vi "SortGraphIndex.vi"(4 "Error In":errorcluster, 7 "ConfigurationTotale":T2) -> (0 "Error Out":errorcluster, 3 "GraphIndex":T1)   [LabVIEW 2017]
uses:
  DefDeType/ConfigTotale.ctl
  DefDeType/VoltageChannels.ctl
  DefDeType/WBridgeChannels.ctl
  DefDeType/Configuration.ctl
panel:
  out "Graph2Indexes":i32[](array[numeric])
  out "Graph1Indexes":i32[](array[numeric])
  out "appended array":u8[](array[numeric])
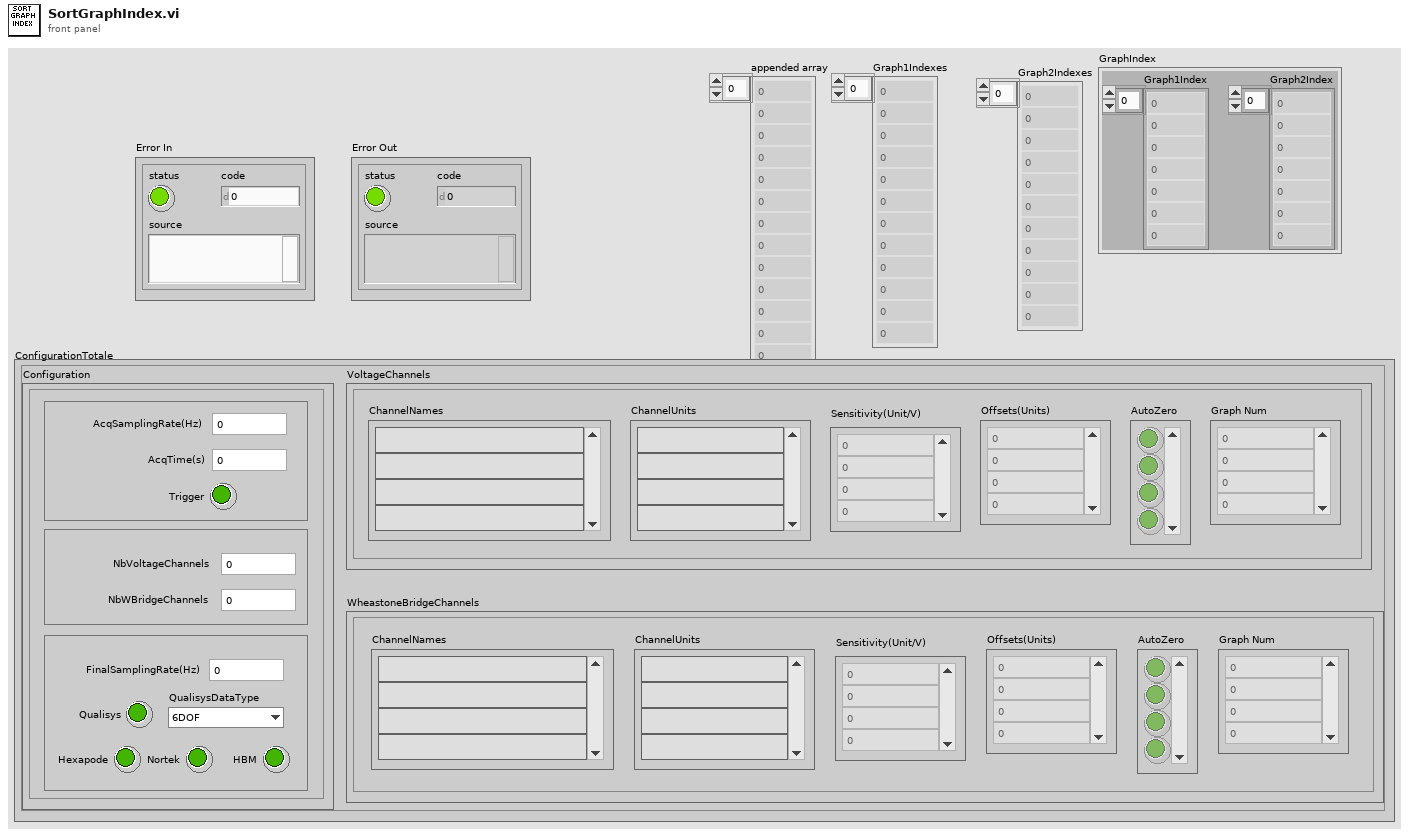
[diagram p1: front panel]
types:
  T1 = cluster{"Graph2Index":i32[], "Graph1Index":i32[]}
  T2 = typedef "ConfigTotale.ctl" = cluster{"VoltageChannels":T3, "WheastoneBridgeChannels":T4, "Configuration":T5}
  T3 = typedef "VoltageChannels.ctl" = cluster{"ChannelNames":string[], "Sensitivity(Unit/V)":dbl[], "AutoZero":bool[], "ChannelUnits":string[], "Offsets(Units)":dbl[], "Graph Num":u8[]}
  T4 = typedef "WBridgeChannels.ctl" = cluster{"ChannelNames":string[], "Sensitivity(Unit/V)":dbl[], "AutoZero":bool[], "ChannelUnits":string[], "Offsets(Units)":dbl[], "Graph Num":u8[]}
  T5 = typedef "Configuration.ctl" = cluster{"AcqSamplingRate(Hz)":u32, "AcqTime(s)":u32, "Trigger":bool, "NbVoltageChannels":u32, "NbWBridgeChannels":u32, "Qualisys":bool, "Hexapode":bool, "FinalSamplingRate(Hz)":u32, "QualisysDataType":enum16{"6DOF", "3DTracking", "6DOF + 3D"}, "Nortek":bool, "HBM":bool}
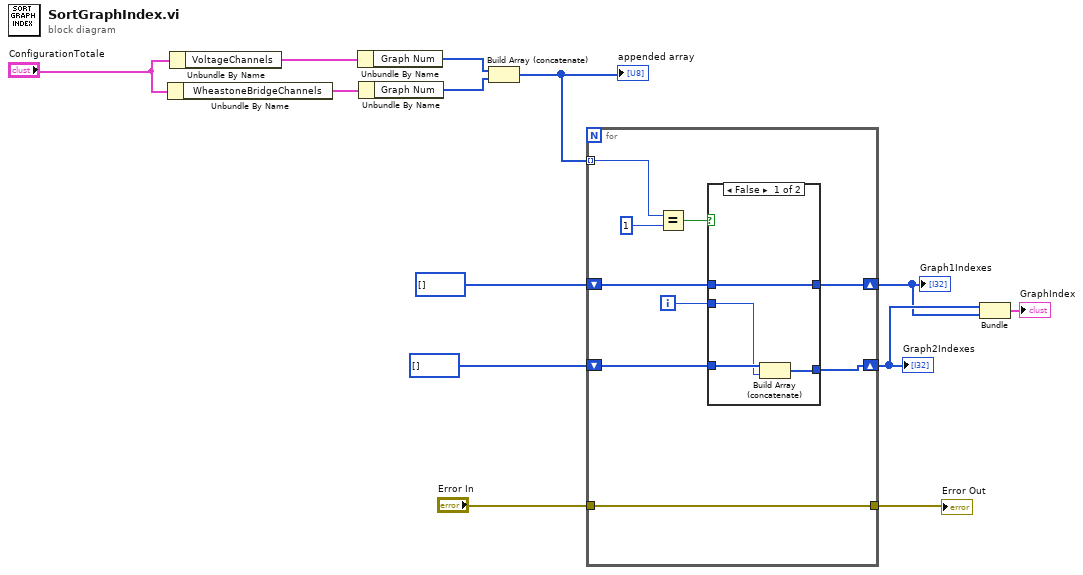
[diagram p0: block diagram]
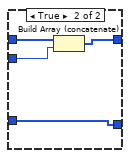
[diagram p2: hidden frame]
diagram:
  n1 = Unbundle By Name("ConfigurationTotale") -> ("WheastoneBridgeChannels"=w12:T4)
  n2 = Unbundle By Name("ConfigurationTotale") -> ("VoltageChannels"=w13:T3)
  n3 = Unbundle By Name(w13) -> ("Graph Num"=w11:u8[])
  n4 = Unbundle By Name(w12) -> ("Graph Num"=w10:u8[])
  n5 = Build Array (concatenate)(w11, w10) -> (w8:u8[])
  "appended array" <- w8
  n6 = for {
    tunnel: w8 -> [w22] mode=indexing
    shift-right: [w18] -> w1
    shift-left: i32[] [] -> [w19]
    shift-right: [w15] -> w2
    shift-left: i32[] [] -> [w16]
    tunnel: [w14] -> w4
    tunnel: "Error In" -> [w14]
    i -> [w17]
    n7 = Equal?(x=w22, y=u8 1) -> (x = y?=w20:bool)
    n8 = case shown="False" w20 {
      tunnel: w19 -> [w26 w30]
      tunnel: [w26 w29] -> w18
      tunnel: w17 -> [w24 w28]
      tunnel: w16 -> [w25 w27]
      tunnel: [w23 w27] -> w15
      frame False {
        n9 = Build Array (concatenate)(w25, w24) -> (w23:i32[])
      }
      frame True {
        n10 = Build Array (concatenate)(w30, w28) -> (w29:i32[])
      }
    }
  }
  "Graph1Indexes" <- w1
  "Graph2Indexes" <- w2
  "Error Out" <- w4
  n11 = Bundle(w2, w1) -> (→"GraphIndex":cluster{i32[], i32[]})  [unwired: 1 in]
